vi "WriteDashValues.vi"(8 "error in (no error)":errorcluster, 10 "output cluster":T1) -> (0 "error out":errorcluster)   [LabVIEW 2014]
uses:
  buttons/PresetValues.ctl
  <vilib>/Utility/config.llb/Write Key (Double).vi
  <vilib>/Utility/config.llb/NI_LVConfig.lvlib
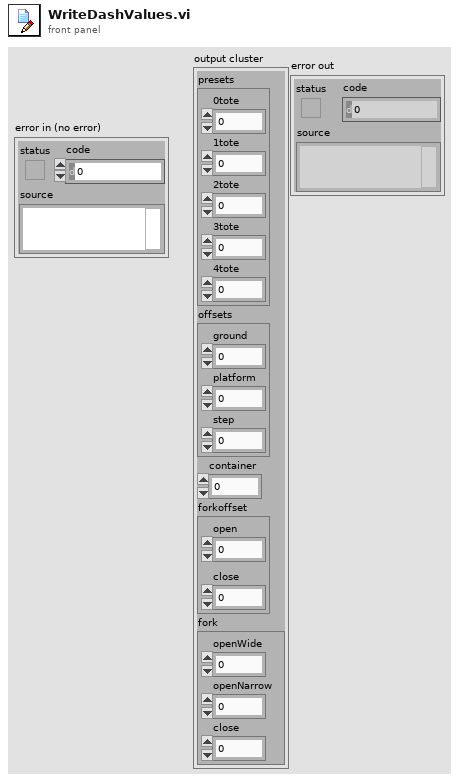
[diagram p1: front panel]
types:
  T1 = typedef "PresetValues.ctl" = cluster{"presets":cluster{"0tote":dbl, "1tote":dbl, "2tote":dbl, "3tote":dbl, "4tote":dbl}, "offsets":cluster{"ground":dbl, "platform":dbl, "step":dbl}, "container":dbl, "forkoffset":cluster{"open":dbl, "close":dbl}, "fork":cluster{"openWide":dbl, "openNarrow":dbl, "close":dbl}}
  T2 = typedef "NI_LVConfig.lvlib/Config Data RefNum.ctl" = refnum<k1>
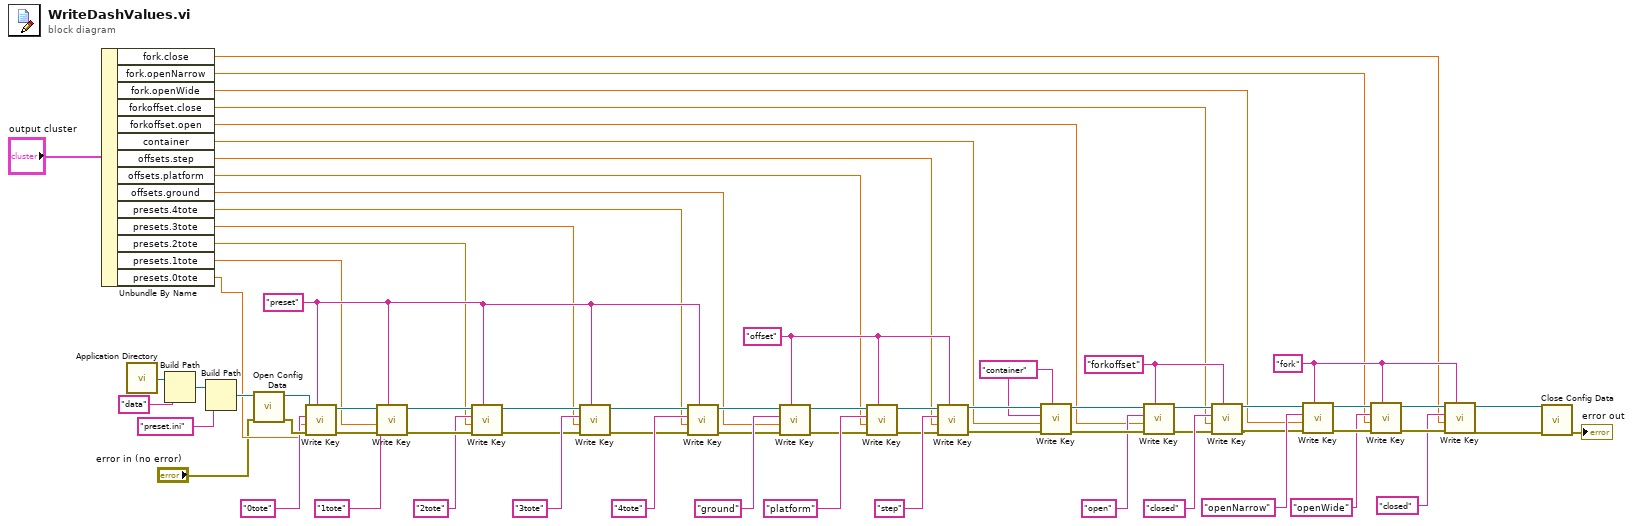
[diagram p0: block diagram]
diagram:
  w23 = "fork" ("section")
  w31 = "forkoffset" ("section")
  w39 = "container" ("section")
  w48 = "offset" ("section")
  w50 = "preset" ("section")
  n1 = Unbundle By Name("output cluster") -> ("fork.close"=w3:dbl, "fork.openNarrow"=w4:dbl, "fork.openWide"=w5:dbl, "forkoffset.close"=w6:dbl, "forkoffset.open"=w7:dbl, "container"=w8:dbl, "offsets.step"=w9:dbl, "offsets.platform"=w10:dbl, "offsets.ground"=w11:dbl, "presets.4tote"=w12:dbl, "presets.3tote"=w13:dbl, "presets.2tote"=w14:dbl, "presets.1tote"=w16:dbl, "presets.0tote"=w17:dbl)
  n2 = call <vilib>:"Application Directory.vi"() -> ("Application Directory"=w67:path)
  n3 = Build Path(base path=w67, name or relative path="data") -> (appended path=w65:path)
  n4 = Build Path(base path=w65, name or relative path="preset.ini") -> (appended path=w63:path)
  n5 = call <vilib>:"Open Config Data.vi"("error in (no error)"="error in (no error)", "configuration file path"=w63) -> ("error out"=w70:errorcluster, "refnum"=w69:T2)  [unwired: 7 in, 1 out]
  n6 = call-poly <vilib>:"Write Key.vi"("section"=w50, "error in (no error)"=w70, "value"=w17, "key"="0tote", "refnum"=w69) -> ("error out"=w46:errorcluster, "refnum out"=w62:T2)  [unwired: 4 in, 1 out]
  n7 = call-poly <vilib>:"Write Key.vi"("section"=w50, "error in (no error)"=w46, "value"=w16, "key"="1tote", "refnum"=w62) -> ("error out"=w45:errorcluster, "refnum out"=w60:T2)  [unwired: 4 in, 1 out]
  n8 = call-poly <vilib>:"Write Key.vi"("section"=w50, "error in (no error)"=w45, "value"=w14, "key"="2tote", "refnum"=w60) -> ("error out"=w44:errorcluster, "refnum out"=w59:T2)  [unwired: 4 in, 1 out]
  n9 = call-poly <vilib>:"Write Key.vi"("section"=w50, "error in (no error)"=w44, "value"=w13, "key"="3tote", "refnum"=w59) -> ("error out"=w43:errorcluster, "refnum out"=w57:T2)  [unwired: 4 in, 1 out]
  n10 = call-poly <vilib>:"Write Key.vi"("section"=w50, "error in (no error)"=w43, "value"=w12, "key"="4tote", "refnum"=w57) -> ("error out"=w42:errorcluster, "refnum out"=w55:T2)  [unwired: 4 in, 1 out]
  n11 = call-poly <vilib>:"Write Key.vi"("section"=w48, "error in (no error)"=w42, "value"=w11, "key"="ground", "refnum"=w55) -> ("error out"=w41:errorcluster, "refnum out"=w54:T2)  [unwired: 4 in, 1 out]
  n12 = call-poly <vilib>:"Write Key.vi"("section"=w48, "error in (no error)"=w41, "value"=w10, "key"="platform", "refnum"=w54) -> ("error out"=w40:errorcluster, "refnum out"=w51:T2)  [unwired: 4 in, 1 out]
  n13 = call-poly <vilib>:"Write Key.vi"("section"=w48, "error in (no error)"=w40, "value"=w9, "key"="step", "refnum"=w51) -> ("error out"=w38:errorcluster, "refnum out"=w47:T2)  [unwired: 4 in, 1 out]
  n14 = call-poly <vilib>:"Write Key.vi"("section"=w39, "error in (no error)"=w38, "value"=w8, "key"=w39, "refnum"=w47) -> ("error out"=w36:errorcluster, "refnum out"=w37:T2)  [unwired: 4 in, 1 out]
  n15 = call-poly <vilib>:"Write Key.vi"("section"=w31, "error in (no error)"=w36, "value"=w7, "key"="open", "refnum"=w37) -> ("error out"=w34:errorcluster, "refnum out"=w33:T2)  [unwired: 4 in, 1 out]
  n16 = call-poly <vilib>:"Write Key.vi"("section"=w31, "error in (no error)"=w34, "value"=w6, "key"="closed", "refnum"=w33) -> ("error out"=w25:errorcluster, "refnum out"=w26:T2)  [unwired: 4 in, 1 out]
  n17 = call-poly <vilib>:"Write Key.vi"("section"=w23, "error in (no error)"=w25, "value"=w5, "key"="openNarrow", "refnum"=w26) -> ("error out"=w28:errorcluster, "refnum out"=w29:T2)  [unwired: 4 in, 1 out]
  n18 = call-poly <vilib>:"Write Key.vi"("section"=w23, "error in (no error)"=w28, "value"=w4, "key"="openWide", "refnum"=w29) -> ("error out"=w20:errorcluster, "refnum out"=w24:T2)  [unwired: 4 in, 1 out]
  n19 = call-poly <vilib>:"Write Key.vi"("section"=w23, "error in (no error)"=w20, "value"=w3, "key"="closed", "refnum"=w24) -> ("error out"=w21:errorcluster, "refnum out"=w22:T2)  [unwired: 4 in, 1 out]
  n20 = call <vilib>:"Close Config Data.vi"("error in (no error)"=w21, "refnum"=w22) -> ("error out"=→"error out":errorcluster)  [unwired: 8 in, 1 out]
